vi "Write Controller.vi"(8 "error in (no error)":errorcluster, 10 "UIContainer.lvlib:Controller.lvclass":refnum<class "Controller.lvclass">, 11 "View in":refnum<class "View.lvclass">) -> (0 "error out":errorcluster, 3 "View out":refnum<class "View.lvclass">)   [LabVIEW 2020, in "UIContainer.lvlib" / "View.lvclass"]
uses:
  View.lvclass
  View.lvclass/View.ctl
  Controller/Controller.lvclass
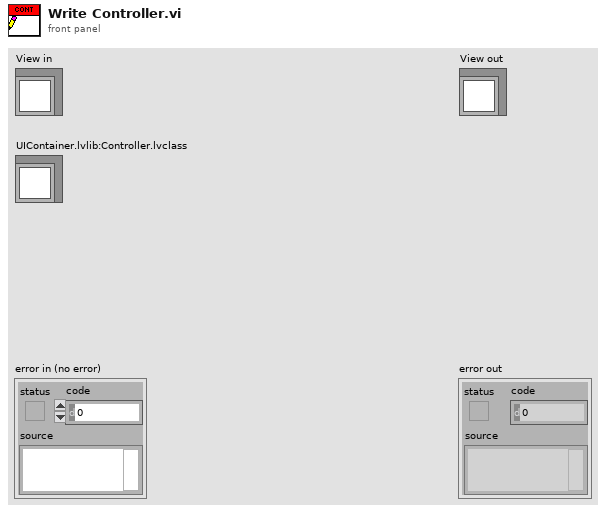
[diagram p1: front panel]
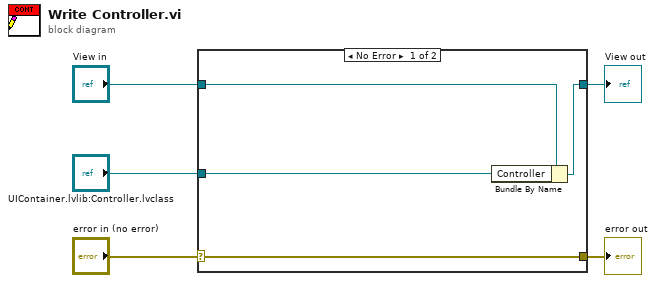
[diagram p0: block diagram]
diagram:
  n1 = case shown="No Error" "error in (no error)" {
    selector: "error in (no error)" -> [w9 w10]
    tunnel: [w9 w10] -> w4
    tunnel: [w7 w11] -> w2
    tunnel: "View in" -> [w8 w11]
    tunnel: "UIContainer.lvlib:Controller.lvclass" -> [w6 _]
    frame No Error {
      n2 = Bundle By Name(cluster=w8, "Controller"=w6) -> (w7:refnum<class "View.lvclass">)
    }
    frame Error {
    }
  }
  "error out" <- w4
  "View out" <- w2
